vi "polarPlotData.vi"(7 "reset":bool, 11 "hits":T1[](array[typedef])) -> (3 "polar_plot_data":T2[](array[typedef]))   [LabVIEW 2018]
uses:
  polar_data.ctl
  AE/hit_data.ctl
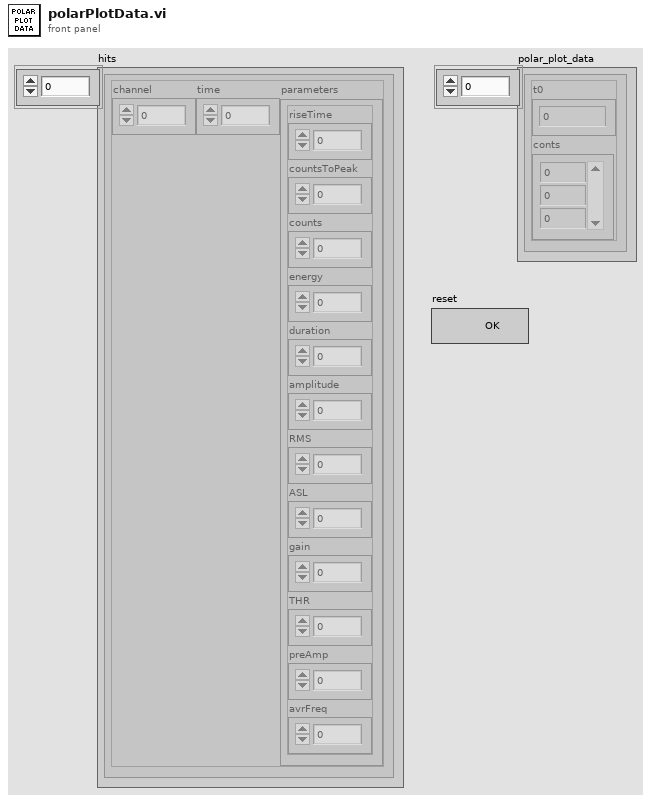
[diagram p1: front panel]
types:
  T1 = typedef "hit_data.ctl" = cluster{"channel":u8, "time":dbl, "parameters":cluster{"riseTime":u32, "countsToPeak":u32, "counts":u32, "energy":u32, "duration":u32, "amplitude":u32, "RMS":u32, "ASL":u32, "gain":u32, "THR":u32, "preAmp":u32, "avrFreq":u32}}
  T2 = typedef "polar_data.ctl" = cluster{"t0":dbl, "conts":dbl[]}
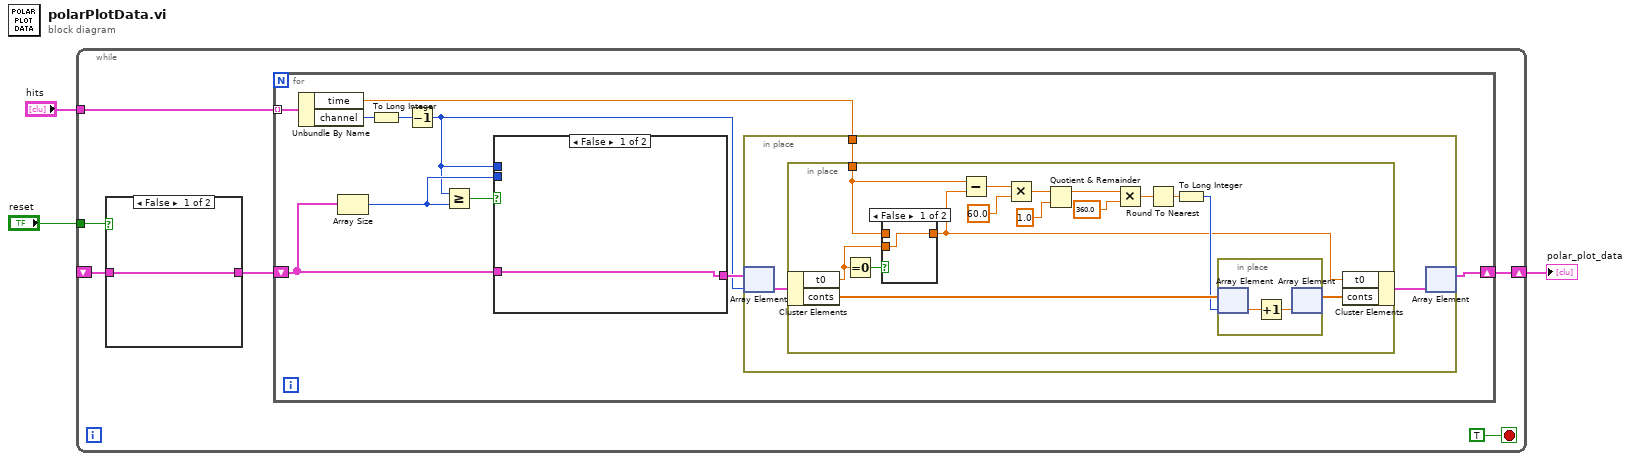
[diagram p0: block diagram]
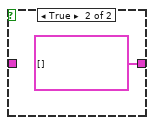
[diagram p2: hidden frame]
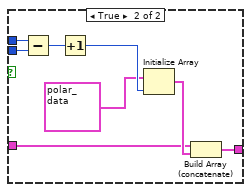
[diagram p3: hidden frame]
diagram:
  n1 = while {
    tunnel: "hits" -> [w8]
    shift-right: [w9] -> w3
    shift-left: _ -> [w5]
    tunnel: "reset" -> [w6]
    stop <- TRUE stop-if-true
    n2 = case shown="False" w6 {
      tunnel: w5 -> [w10 _]
      tunnel: [w10 T2[] []] -> w4
      frame False {
      }
      frame True {
      }
    }
    n3 = for {
      tunnel: w8 -> [w21] mode=indexing
      shift-right: [w14] -> w9
      shift-left: w4 -> [w17]
      n4 = Unbundle By Name(w21) -> ("time"=w13:dbl, "channel"=w20:u8)
      n5 = Array Size(array=w17) -> (size(s)=w18:i32)
      n6 = To Long Integer(number=w20) -> (32bit integer=w12:i32)
      n7 = Decrement(x=w12) -> (x-1=w15:i32)
      n8 = Greater Or Equal?(x=w15, y=w18) -> (x >= y?=w19:bool)
      n9 = case shown="False" w19 {
        tunnel: w15 -> [_ w30]
        tunnel: w18 -> [_ w29]
        tunnel: w17 -> [w22 w25]
        tunnel: [w22 w24] -> w16
        frame False {
        }
        frame True {
          n10 = Subtract(x=w30, y=w29) -> (x-y=w28:i32)
          n11 = Increment(x=w28) -> (x+1=w27:i32)
          n12 = Initialize Array(T2 {"t0"=0.0, "conts"=[0.0, 0.0, 0.0, 0.0, 0.0, 0.0, 0.0, 0.0, 0.0, 0.0, 0.0, 0.0, 0.0, 0.0, 0.0, 0.0, 0.0, 0.0, 0.0, 0.0, 0.0, 0.0, 0.0, 0.0, 0.0, 0.0, 0.0, 0.0, 0.0, 0.0, 0.0, 0.0, 0.0, 0.0, 0.0, 0.0, 0.0, 0.0, 0.0, 0.0, 0.0, 0.0, 0.0, 0.0, 0.0, 0.0, 0.0, 0.0, 0.0, 0.0, 0.0, 0.0, 0.0, 0.0, 0.0, 0.0, 0.0, 0.0, 0.0, 0.0, 0.0, 0.0, 0.0, 0.0, 0.0, 0.0, 0.0, 0.0, 0.0, 0.0, 0.0, 0.0, 0.0, 0.0, 0.0, 0.0, 0.0, 0.0, 0.0, 0.0, 0.0, 0.0, 0.0, 0.0, 0.0, 0.0, 0.0, 0.0, 0.0, 0.0, 0.0, 0.0, 0.0, 0.0, 0.0, 0.0, 0.0, 0.0, 0.0, 0.0, 0.0, 0.0, 0.0, 0.0, 0.0, 0.0, 0.0, 0.0, 0.0, 0.0, 0.0, 0.0, 0.0, 0.0, 0.0, 0.0, 0.0, 0.0, 0.0, 0.0, 0.0, 0.0, 0.0, 0.0, 0.0, 0.0, 0.0, 0.0, 0.0, 0.0, 0.0, 0.0, 0.0, 0.0, 0.0, 0.0, 0.0, 0.0, 0.0, 0.0, 0.0, 0.0, 0.0, 0.0, 0.0, 0.0, 0.0, 0.0, 0.0, 0.0, 0.0, 0.0, 0.0, 0.0, 0.0, 0.0, 0.0, 0.0, 0.0, 0.0, 0.0, 0.0, 0.0, 0.0, 0.0, 0.0, 0.0, 0.0, 0.0, 0.0, 0.0, 0.0, 0.0, 0.0, 0.0, 0.0, 0.0, 0.0, 0.0, 0.0, 0.0, 0.0, 0.0, 0.0, 0.0, 0.0, 0.0, 0.0, 0.0, 0.0, 0.0, 0.0, 0.0, 0.0, 0.0, 0.0, 0.0, 0.0, 0.0, 0.0, 0.0, 0.0, 0.0, 0.0, 0.0, 0.0, 0.0, 0.0, 0.0, 0.0, 0.0, 0.0, 0.0, 0.0, 0.0, 0.0, 0.0, 0.0, 0.0, 0.0, 0.0, 0.0, 0.0, 0.0, 0.0, 0.0, 0.0, 0.0, 0.0, 0.0, 0.0, 0.0, 0.0, 0.0, 0.0, 0.0, 0.0, 0.0, 0.0, 0.0, 0.0, 0.0, 0.0, 0.0, 0.0, 0.0, 0.0, 0.0, 0.0, 0.0, 0.0, 0.0, 0.0, 0.0, 0.0, 0.0, 0.0, 0.0, 0.0, 0.0, 0.0, 0.0, 0.0, 0.0, 0.0, 0.0, 0.0, 0.0, 0.0, 0.0, 0.0, 0.0, 0.0, 0.0, 0.0, 0.0, 0.0, 0.0, 0.0, 0.0, 0.0, 0.0, 0.0, 0.0, 0.0, 0.0, 0.0, 0.0, 0.0, 0.0, 0.0, 0.0, 0.0, 0.0, 0.0, 0.0, 0.0, 0.0, 0.0, 0.0, 0.0, 0.0, 0.0, 0.0, 0.0, 0.0, 0.0, 0.0, 0.0, 0.0, 0.0, 0.0, 0.0, 0.0, 0.0, 0.0, 0.0, 0.0, 0.0, 0.0, 0.0, 0.0, 0.0, 0.0, 0.0, 0.0, 0.0, 0.0, 0.0, 0.0, 0.0, 0.0, 0.0, 0.0, 0.0, 0.0, 0.0, 0.0, 0.0, 0.0, 0.0, 0.0, 0.0, 0.0, 0.0, 0.0, 0.0, 0.0, 0.0, 0.0, 0.0, 0.0, 0.0, 0.0, 0.0, 0.0, 0.0, 0.0, 0.0, 0.0]} ("output cluster"), w27) -> (w26:T2[])
          n13 = Build Array (concatenate)(w25, w26) -> (w24:T2[])
        }
      }
      n14 = in-place {
        in-place-border: w13 -> [w31]
        n15 = in-place-array #1(w16, w15) -> (w33:T2)
        n16 = in-place {
          in-place-border: w31 -> [w41]
          n17 = in-place-cluster #2(w33) -> ("t0"=w45:dbl, "conts"=w48:dbl[])
          n18 = Equal To 0?(x=w45) -> (x = 0?=w46:bool)
          n19 = case shown="False" w46 {
            tunnel: w41 -> [_ w50]
            tunnel: w45 -> [w49 _]
            tunnel: [w49 w50] -> w34
            frame False {
            }
            frame True {
            }
          }
          n20 = Subtract(x=w41, y=w34) -> (x-y=w37:dbl)
          n21 = Multiply(x=w37, y=60.0 ("x")) -> (x*y=w35:dbl)
          n22 = Quotient & Remainder(x=w35, y=1.0) -> (x-y*floor(x/y)=w42:dbl)  [unwired: 1 out]
          n23 = Multiply(x=w42, y=360.0) -> (x*y=w44:dbl)
          n24 = Round To Nearest(number=w44) -> (nearest integer value=w38:dbl)
          n25 = To Long Integer(number=w38) -> (32bit integer=w40:i32)
          n26 = in-place {
            n27 = in-place-array #3(w48, w40) -> (w52:dbl)
            n28 = Increment(x=w52) -> (x+1=w51:dbl)
            n29 = in-place-array #3(w51) -> (w47:dbl[])  [unwired: 1 out]
          }
          n30 = in-place-cluster #2("t0"=w34, "conts"=w47) -> (w32:T2)
        }
        n31 = in-place-array #1(w32) -> (w14:T2[])  [unwired: 1 out]
      }
    }
  }
  "polar_plot_data" <- w3
